vi "4xMonitor.vi"   [LabVIEW 2016]
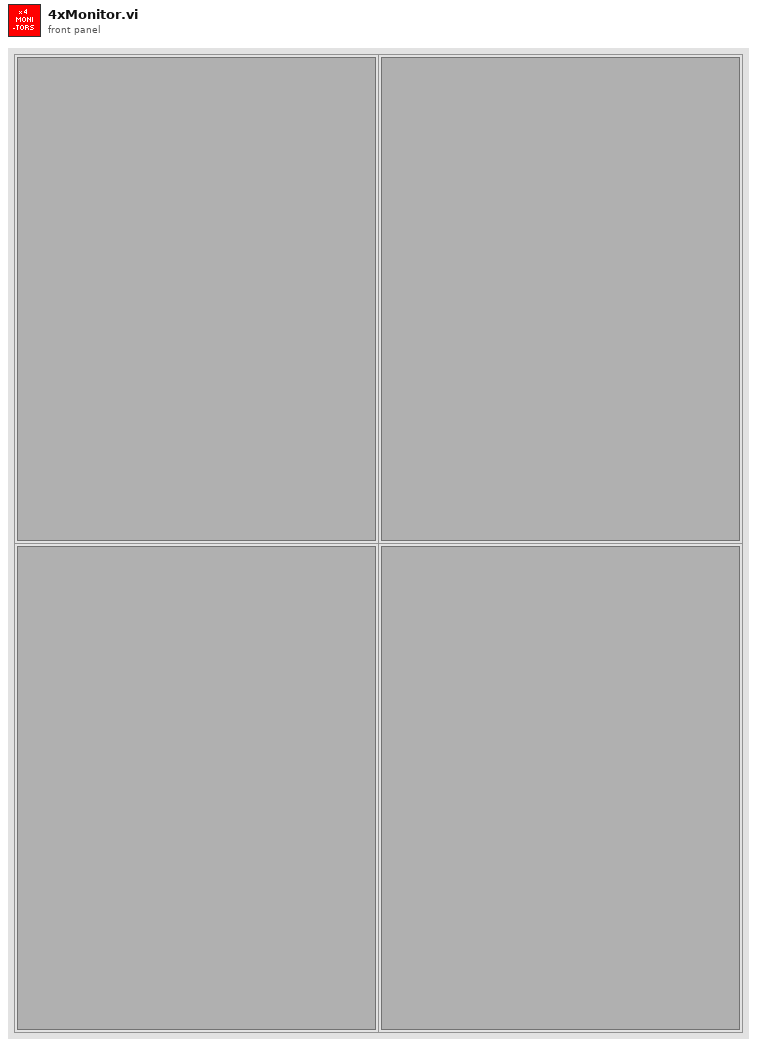
[diagram p1: front panel]
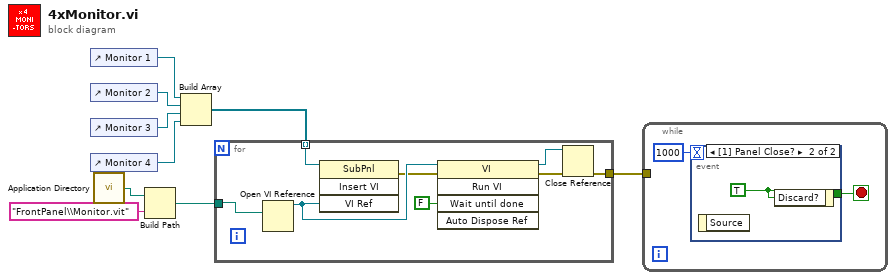
[diagram p0: block diagram]
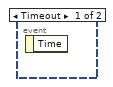
[diagram p2: hidden frame]
diagram:
  n1 = control-ref of="Monitor 1"() -> (w6:refnum<vi>)
  n2 = control-ref of="Monitor 2"() -> (w5:refnum<vi>)
  n3 = control-ref of="Monitor 3"() -> (w4:refnum<vi>)
  n4 = control-ref of="Monitor 4"() -> (w3:refnum<vi>)
  n5 = call <vilib>:"Application Directory.vi"() -> ("Application Directory"=w9:path)
  n6 = Build Path(base path=w9, name or relative path="FrontPanel\\Monitor.vit") -> (appended path=w8:path)
  n7 = Build Array(w6, w5, w4, w3) -> (w2:refnum<vi>[])
  n8 = for {
    tunnel: w8 -> [w13]
    tunnel: w2 -> [w17] mode=indexing
    tunnel: [w10] -> w1
    n9 = Open VI Reference(vi path=w13) -> (vi reference=w16:refnum<vi>)  [unwired: 5 in, 1 out]
    n10 = invoke on="Invoke Node" class="SubPnl" method="Insert VI"(reference=w17, "VI Ref"=w16) -> (error out=w15:errorcluster)  [unwired: 2 in, 3 out]
    n11 = invoke class="VI" method="Run VI"(reference=w16, error in=w15, "Wait until done"=FALSE ("Wait Until Done")) -> (reference out=w12:refnum<vi>, error out=w11:errorcluster)  [unwired: 2 in, 3 out]
    n12 = Close Reference(reference=w12, error in (no error)=w11) -> (error out=w10:errorcluster)
  }
  n13 = while {
    tunnel: w1 -> [_]
    stop <- w19 stop-if-true
    n14 = event shown="[1] Panel Close?" {
      selector: _ -> [_ _]
      dyn-events: _ -> [_ _]
      timeout: 1000 -> [_ _]
      tunnel: [_ w20] -> w19
      event Timeout {
        n15 = event-data() -> ()  [unwired: 1 in, 1 out]
      }
      event Panel Close? {
        w20 = TRUE ("stop")
        n16 = event-data() -> ()  [unwired: 1 in, 1 out]
        n17 = event-data("Discard?"=w20) -> ()  [unwired: 1 in, 1 out]
      }
    }
  }
